vi "单通道转换scan list.vi"(1 "测量通道数":i32=2 min=1 max=100) -> (0 "Scan List":string)   [LabVIEW 2015]
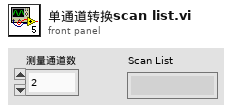
[diagram p1: front panel]
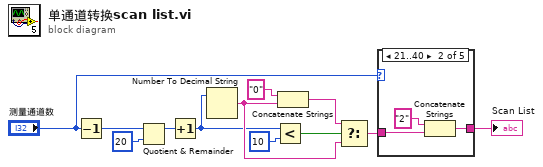
[diagram p0: block diagram]
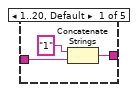
[diagram p2: hidden frame]
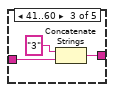
[diagram p3: hidden frame]
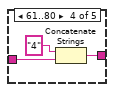
[diagram p4: hidden frame]
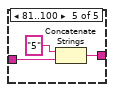
[diagram p5: hidden frame]
diagram:
  n1 = Decrement(x="测量通道数") -> (x-1=w3:i32)
  n2 = Quotient & Remainder(x=w3, y=20) -> (x-y*floor(x/y)=w8:i32)  [unwired: 1 out]
  n3 = Increment(x=w8) -> (x+1=w1:i32)
  n4 = Number To Decimal String(number=w1) -> (decimal integer string=w6:string)  [unwired: 1 in]
  n5 = Less?(x=w1, y=10) -> (x < y?=w10:bool)
  n6 = Concatenate Strings("0" ("Scan List"), w6) -> (w7:string)
  n7 = Select(t=w7, s=w10, f=w6) -> (s? t:f=w5:string)
  n8 = case shown="21..40" "测量通道数" {
    tunnel: w5 -> [w15 w18 w21 w24 w27]
    tunnel: [w13 w16 w19 w22 w25] -> w4
    frame 1..20, Default {
      n9 = Concatenate Strings("1" ("Scan List"), w15) -> (w13:string)
    }
    frame 21..40 {
      n10 = Concatenate Strings("2" ("Scan List"), w18) -> (w16:string)
    }
    frame 41..60 {
      n11 = Concatenate Strings("3" ("Scan List"), w21) -> (w19:string)
    }
    frame 61..80 {
      n12 = Concatenate Strings("4" ("Scan List"), w24) -> (w22:string)
    }
    frame 81..100 {
      n13 = Concatenate Strings("5" ("Scan List"), w27) -> (w25:string)
    }
  }
  "Scan List" <- w4
